vi "Bar Code Reader_v2.vi"() -> ()   [LabVIEW 2016]
uses:
  <vilib>/NXT/Dual Mode Library/Sensors/EV3_Color_Color.vi
  <vilib>/NXT/NXTIO Xnodes/NXTIONodeSubVIs/LEGOMoveAllMotors.vi
  <vilib>/NXT/NXTIO Xnodes/NXTIONodeSubVIs/LEGOMoveAllMotorsDistance.vi
  <vilib>/NXT/Subs/LVHSConnector.ctl
  <vilib>/NXT/NXTIO Xnodes/NXTIOXNode/NXTIO.xnode
  <vilib>/NXT/LegoClasses/BrickReference/BrickReference.lvclass
panel:
  out "Type 2":dbl
  out "Type 1":dbl
  out "String 3":string
  out "String 2":string
  out "Material":string
  out "String":string
  out "Numeric":dbl
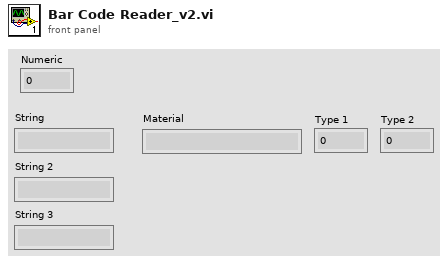
[diagram p1: front panel]
types:
  T1 = typedef "ColorSensorColors.ctl" = enum16{"No Color", "Black", "Blue", "Green", "Yellow", "Red", "White", "Brown"}
  T2 = typedef "LVHSConnector.ctl" = refnum<class "BrickReference.lvclass">
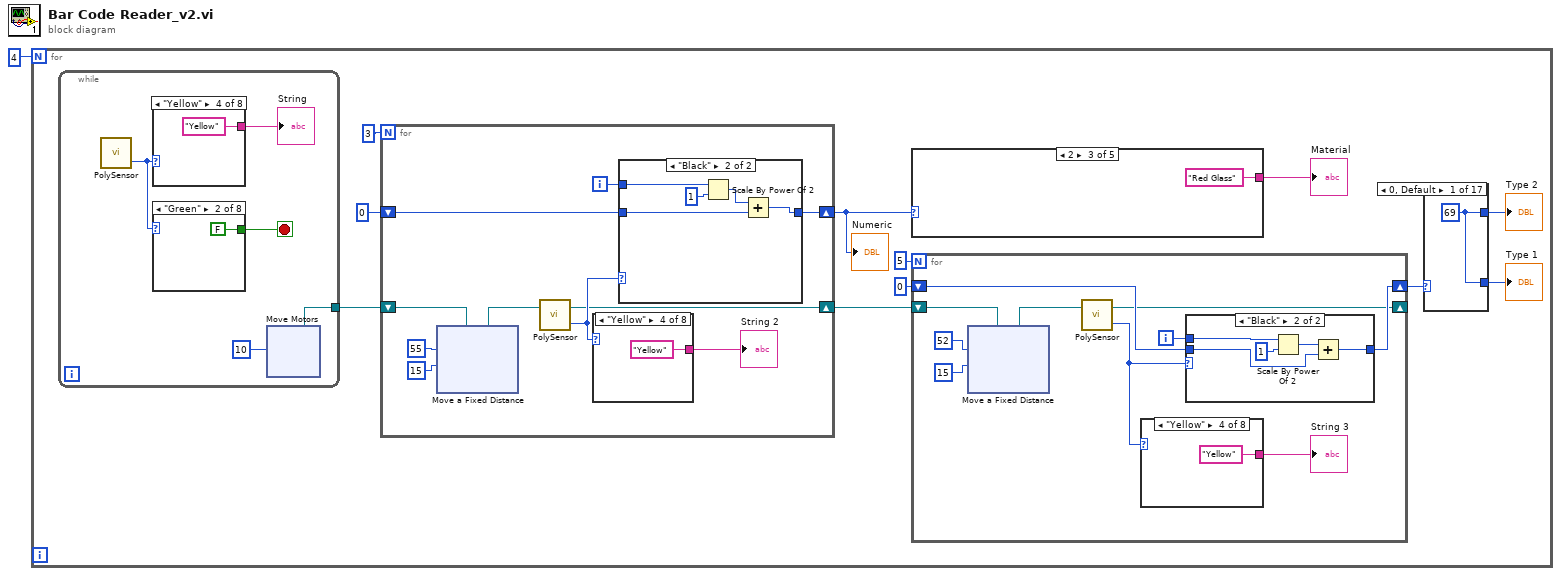
[diagram p0: block diagram]
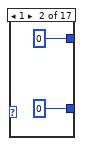
[diagram p2: hidden frame]
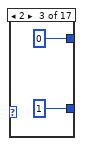
[diagram p3: hidden frame]
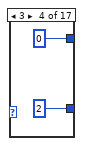
[diagram p4: hidden frame]
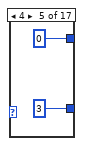
[diagram p5: hidden frame]
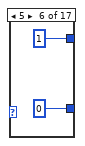
[diagram p6: hidden frame]
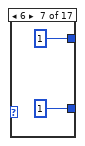
[diagram p7: hidden frame]
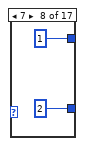
[diagram p8: hidden frame]
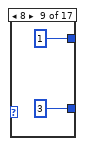
[diagram p9: hidden frame]
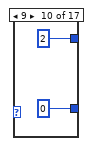
[diagram p10: hidden frame]
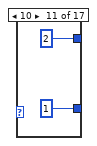
[diagram p11: hidden frame]
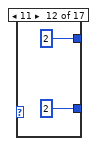
[diagram p12: hidden frame]
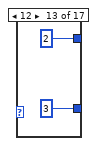
[diagram p13: hidden frame]
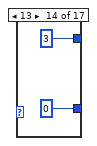
[diagram p14: hidden frame]
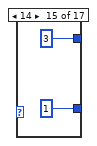
[diagram p15: hidden frame]
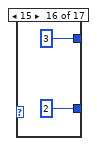
[diagram p16: hidden frame]
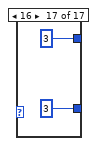
[diagram p17: hidden frame]
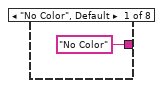
[diagram p18: hidden frame]
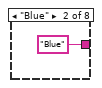
[diagram p19: hidden frame]
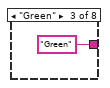
[diagram p20: hidden frame]
diagram:
  n1 = for {
    N: 4 -> [_]
    n2 = while {
      tunnel: [w83] -> w2
      stop <- w86 stop-if-true
      n3 = call-poly <vilib>:"PolySensor.vi"() -> ("Detected Color"=w84:T1)  [unwired: 3 in, 1 out]
      n4 = case shown="\"Yellow\"" w84 {
        tunnel: ["No Color" "Blue" "Green" "Yellow" "Red" "White" "Brown" "Black"] -> w85
        frame "No Color", Default {
        }
        frame "Blue" {
        }
        frame "Green" {
        }
        frame "Yellow" {
        }
        frame "Red" {
        }
        frame "White" {
        }
        frame "Brown" {
        }
        frame "Black" {
        }
      }
      "String" <- w85
      n5 = case shown="\"Green\"" w84 {
        tunnel: [FALSE FALSE FALSE FALSE FALSE FALSE FALSE TRUE] -> w86
        frame "No Color", Default {
        }
        frame "Green" {
        }
        frame "Yellow" {
        }
        frame "Red" {
        }
        frame "White" {
        }
        frame "Brown" {
        }
        frame "Blue" {
        }
        frame "Black" {
        }
      }
      n6 = xnode "Move Motors"("Power/Speed 1"=i8 10) -> ("NXT/EV3"=w83:T2)  [unwired: 2 in]
    }
    n7 = for {
      N: 3 -> [_]
      shift-right: [w117] -> w10
      shift-left: 0 -> [w116]
      shift-right: [w112] -> w6
      shift-left: w2 -> [w111]
      i -> [w113]
      n8 = xnode "Move a Fixed Distance"("Speed 1"=i8 15, "Distance 1"=55, "NXT/EV3"=w111) -> ("NXT/EV3"=w110:T2)  [unwired: 1 in]
      n9 = call-poly <vilib>:"PolySensor.vi"("NXT/EV3"=w110) -> ("Detected Color"=w114:T1, "NXT/EV3"=w112:T2)  [unwired: 2 in]
      n10 = case shown="\"Yellow\"" w114 {
        tunnel: ["No Color" "Blue" "Green" "Yellow" "Red" "White" "Brown" "Black"] -> w115
        frame "No Color", Default {
        }
        frame "Blue" {
        }
        frame "Green" {
        }
        frame "Yellow" {
        }
        frame "Red" {
        }
        frame "White" {
        }
        frame "Brown" {
        }
        frame "Black" {
        }
      }
      "String 2" <- w115
      n11 = case shown="\"Black\"" w114 {
        tunnel: w113 -> [_ w137]
        tunnel: [w133 w135] -> w117
        tunnel: w116 -> [w133 w134]
        frame "White", Default {
        }
        frame "Black" {
          n12 = Scale By Power Of 2(n=w137, x=1) -> (x*2^n=w136:i32)
          n13 = Add(x=w136, y=w134) -> (x+y=w135:i32)
        }
      }
    }
    "Numeric" <- w10
    n14 = case shown="2" w10 {
      tunnel: ["Something has gone wrong" "White Glass" "Red Glass" "Blue Glass" "Steel/HDPE"] -> w9
      frame 0, Default {
      }
      frame 1 {
      }
      frame 2 {
      }
      frame 3 {
      }
      frame 4 {
      }
    }
    "Material" <- w9
    n15 = for {
      N: 5 -> [_]
      shift-right: [w55] -> w5
      shift-left: 0 -> [w54]
      shift-right: [w50] -> _
      shift-left: w6 -> [w49]
      i -> [w51]
      n16 = xnode "Move a Fixed Distance"("Speed 1"=i8 15, "Distance 1"=52, "NXT/EV3"=w49) -> ("NXT/EV3"=w48:T2)  [unwired: 1 in]
      n17 = call-poly <vilib>:"PolySensor.vi"("NXT/EV3"=w48) -> ("Detected Color"=w52:T1, "NXT/EV3"=w50:T2)  [unwired: 2 in]
      n18 = case shown="\"Yellow\"" w52 {
        tunnel: ["No Color" "Blue" "Green" "Yellow" "Red" "White" "Brown" "Black"] -> w53
        frame "No Color", Default {
        }
        frame "Blue" {
        }
        frame "Green" {
        }
        frame "Yellow" {
        }
        frame "Red" {
        }
        frame "White" {
        }
        frame "Brown" {
        }
        frame "Black" {
        }
      }
      "String 3" <- w53
      n19 = case shown="\"Black\"" w52 {
        tunnel: w51 -> [_ w75]
        tunnel: [w71 w73] -> w55
        tunnel: w54 -> [w71 w72]
        frame "White", Default {
        }
        frame "Black" {
          n20 = Scale By Power Of 2(n=w75, x=1) -> (x*2^n=w74:i32)
          n21 = Add(x=w74, y=w72) -> (x+y=w73:i32)
        }
      }
    }
    n22 = case shown="0, Default" w5 {
      tunnel: [w13 0 1 2 3 0 1 2 3 0 1 2 3 0 1 2 3] -> w4
      tunnel: [w13 0 0 0 0 1 1 1 1 2 2 2 2 3 3 3 3] -> w3
      frame 0, Default {
        w13 = 69
      }
      frame 1 {
      }
      frame 2 {
      }
      frame 3 {
      }
      frame 4 {
      }
      frame 5 {
      }
      frame 6 {
      }
      frame 7 {
      }
      frame 8 {
      }
      frame 9 {
      }
      frame 10 {
      }
      frame 11 {
      }
      frame 12 {
      }
      frame 13 {
      }
      frame 14 {
      }
      frame 15 {
      }
      frame 16 {
      }
    }
    "Type 2" <- w3
    "Type 1" <- w4
  }
